vi "SysInfo-Get Computer Name.vi"() -> (8 "computer name":string)   [LabVIEW 2020]
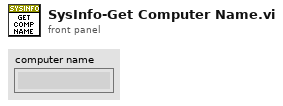
[diagram p1: front panel]
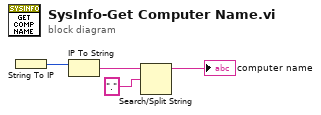
[diagram p0: block diagram]
diagram:
  n1 = String To IP() -> (0:w4:u32)  [unwired: 1 in]
  n2 = IP To String(2:w4) -> (0:w1:string)  [unwired: 1 in]
  n3 = Search/Split String(string=w1, search string/char (-)=".") -> (substring before match=→"computer name":string)  [unwired: 1 in, 2 out]
